vi "Uniform White Noise 2 Points.vi"(0 "amplitude":dbl=1.0 format="%0.2f", 2 "seed":i32, 4 "initialize":bool) -> (5 "uniform white noise 1":dbl format="%0.2f", 6 "uniform white noise 2":dbl format="%0.2f")   [LabVIEW 2017, in "NI_PtbyPt.lvlib"]
uses:
  <vilib>/ptbypt/NI_PtbyPt.lvlib
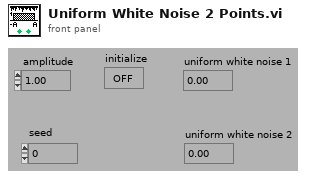
[diagram p1: front panel]
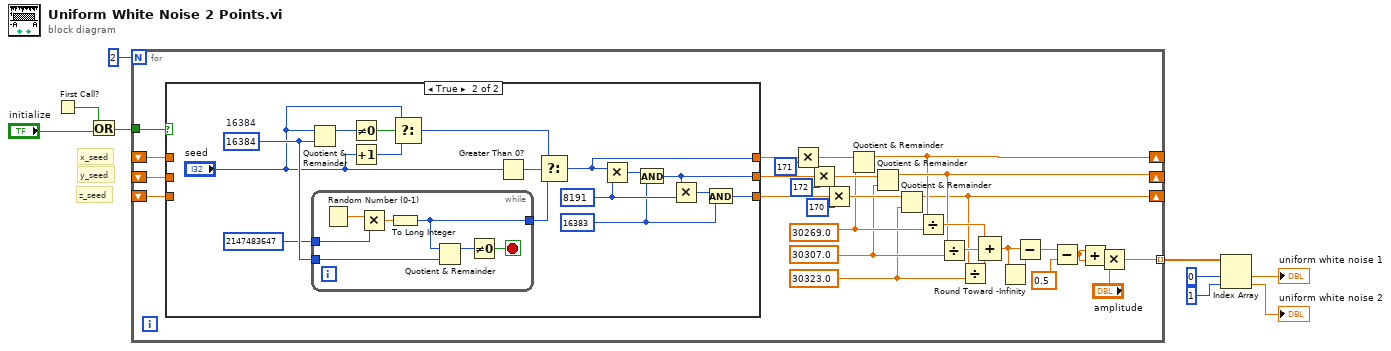
[diagram p0: block diagram]
diagram:
  # "z_seed"
  # "y_seed"
  # "x_seed"
  n1 = First Call?() -> (First Call?: T/F=w8:bool)
  n2 = Or(x=w8, y="initialize") -> (x .or. y?=w7:bool)
  n3 = for {
    N: 2 -> [_]
    shift-right: [w12] -> _
    shift-left: _ -> [w39]
    shift-right: [w13] -> _
    shift-left: _ -> [w38]
    shift-right: [w11] -> _
    shift-left: _ -> [w37]
    tunnel: w7 -> [w19]
    tunnel: [w10] -> w5 mode=indexing
    w20 = 30323.0
    w21 = 30307.0
    w22 = 30269.0
    n4 = case shown="True" w19 {
      tunnel: w39 -> [w42 _]
      tunnel: w38 -> [w41 _]
      tunnel: w37 -> [w40 _]
      tunnel: [w42 w44] -> w36
      tunnel: [w40 w53] -> w35
      tunnel: [w41 w54] -> w34
      frame False {
      }
      frame True {
        w46 = 16384  # 16384
        w56 = 16383
        w58 = 8191 ("y")
        n5 = Quotient & Remainder(x="seed", y=w46) -> (x-y*floor(x/y)=w51:i32)  [unwired: 1 out]
        n6 = while {
          tunnel: [w63] -> w47
          tunnel: w46 -> [w62]
          tunnel: 2147483647 ("x") -> [w59]
          stop <- w60 stop-if-true
          n7 = Random Number (0-1)() -> (number: 0 to 1=w64:dbl)
          n8 = Multiply(x=w64, y=w59) -> (x*y=w65:dbl)
          n9 = To Long Integer(number=w65) -> (32bit integer=w63:i32)
          n10 = Quotient & Remainder(x=w63, y=w62) -> (x-y*floor(x/y)=w61:i32)  [unwired: 1 out]
          n11 = Not Equal To 0?(x=w61) -> (x != 0?=w60:bool)
        }
        n12 = Not Equal To 0?(x=w51) -> (x != 0?=w50:bool)
        n13 = Increment(x="seed") -> (x+1=w49:i32)
        n14 = Select(t="seed", s=w50, f=w49) -> (s? t:f=w48:i32)
        n15 = Greater Than 0?(x="seed") -> (x > 0?=w52:bool)
        n16 = Select(t=w48, s=w52, f=w47) -> (s? t:f=w44:i32)
        n17 = Multiply(x=w44, y=w58) -> (x*y=w55:i32)
        n18 = And(x=w55, y=w56) -> (x .and. y?=w54:i32)
        n19 = Multiply(x=w54, y=w58) -> (x*y=w57:i32)
        n20 = And(x=w57, y=w56) -> (x .and. y?=w53:i32)
      }
    }
    n21 = Multiply(x=w36, y=171) -> (x*y=w23:dbl)
    n22 = Multiply(x=w34, y=172) -> (x*y=w31:dbl)
    n23 = Multiply(x=w35, y=170) -> (x*y=w30:dbl)
    n24 = Quotient & Remainder(x=w23, y=w22) -> (x-y*floor(x/y)=w12:dbl)  [unwired: 1 out]
    n25 = Quotient & Remainder(x=w31, y=w21) -> (x-y*floor(x/y)=w13:dbl)  [unwired: 1 out]
    n26 = Quotient & Remainder(x=w30, y=w20) -> (x-y*floor(x/y)=w11:dbl)  [unwired: 1 out]
    n27 = Divide(x=w12, y=w22) -> (x/y=w29:dbl)
    n28 = Divide(x=w13, y=w21) -> (x/y=w28:dbl)
    n29 = Divide(x=w11, y=w20) -> (x/y=w27:dbl)
    n30 = Compound Arithmetic op=ADD(w29, w28, w27) -> (w26:dbl)
    n31 = Round Toward -Infinity(1:w26) -> (0:w25:dbl)
    n32 = Subtract(x=w26, y=w25) -> (x-y=w17:dbl)
    n33 = Subtract(x=w17, y=0.5) -> (x-y=w14:dbl)
    n34 = Add(x=w14, y=w14) -> (x+y=w15:dbl)
    n35 = Multiply(x=w15, y="amplitude") -> (x*y=w10:dbl)
  }
  n36 = Index Array(array=w5, index #1=0 ("Index"), index #2=1 ("Index")) -> (element #1=→"uniform white noise 1":dbl, element #2=→"uniform white noise 2":dbl)
